vi "DQMH System Message - Removed from Subpanel.vi"(10 "Main VI Path":path) -> (1 "Payload":variant, 2 "Identifier":string="Removed from Subpanel", 5 "Source":T1)   [LabVIEW 2014, in "hse-dqmh.lvlib"]
uses:
  hse-dqmh.lvlib
  Controls/System Message Source.ctl
  Controls/System Message Framework Identifiers.ctl
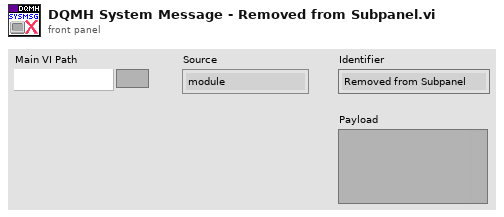
[diagram p1: front panel]
types:
  T1 = typedef "hse-dqmh.lvlib/System Message Source.ctl" = enum16{"module", "application", "network"}
  T2 = typedef "hse-dqmh.lvlib/System Message Framework Identifiers.ctl" = enum16{"Add to Run-Time Menu", "Ready for Display", "Removed from Subpanel"}
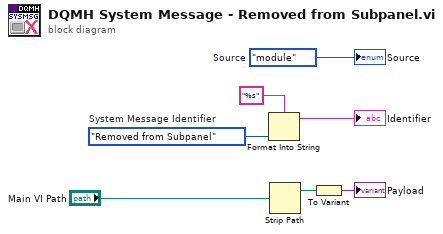
[diagram p0: block diagram]
diagram:
  w5 = System_Message_Framework_Identifiers."Removed from Subpanel"  # System Message Identifier
  w7 = System_Message_Source."module"  # Source
  n1 = Format Into String(format string="%s", w5) -> (resulting string=→"Identifier":string)  [unwired: 2 in, 1 out]
  n2 = Strip Path(path="Main VI Path") -> (stripped path=w2:path)  [unwired: 1 out]
  n3 = To Variant(anything=w2) -> (Variant=→"Payload":variant)
  "Source" <- w7
